vi "number_to_radius.vi"(1 "az":i32) -> (0 "Numeric":i32)   [LabVIEW 2015, in "PolyVIEW.lvclass"]
uses:
  PolyVIEW.lvclass
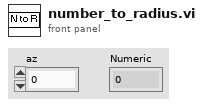
[diagram p1: front panel]
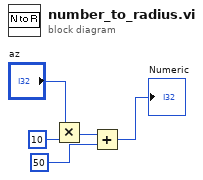
[diagram p0: block diagram]
diagram:
  n1 = Multiply(x="az", y=10) -> (x*y=w2:i32)
  n2 = Add(x=w2, y=50) -> (x+y=→"Numeric":i32)
